vi "Distance elevation and azimuth calculation.vi"(0 "Julian Date":dbl, 2 "Antenna latitude (°)":dbl, 3 "Antenna east longitude (°)":dbl, 4 "Antenna altitude (km)":dbl, 5 "Position Satellite coordinate (ECI)":T1) -> (16 "Azimuth (deg)":dbl, 18 "Elevation (deg)":dbl)   [LabVIEW 2015]
uses:
  <vilib>/Analysis/Matrix/Datatypes/RealMatrix.ctl
  <vilib>/Analysis/Matrix/Numeric/Conversions/Matrix To Array - RM.vi
  Documents/LabVIEW Data/MathScriptVIs/MCStatic_35235434532_9082a658d9e3cba983ee0788969a3ccd.vi
  <instcachedir>/0/MCStatic_35235434532_9082a658d9e3cba983ee0788969a3ccd_E32396614517464C89ABB3D551BA75A9.lvgen/MCStatic_35235434532_9082a658d9e3cba983ee0788969a3ccd_E32396614517464C89ABB3D551BA75A9_000.vi
  Documents/LabVIEW Data/MathScriptVIs/MCStatic_35235434532_d6c4c3a44b84e4e53bab3d751e02fcec.vi
  <instcachedir>/0/MCStatic_35235434532_d6c4c3a44b84e4e53bab3d751e02fcec_188007D13E77446E935A379BA33C246C.lvgen/MCStatic_35235434532_d6c4c3a44b84e4e53bab3d751e02fcec_188007D13E77446E935A379BA33C246C_000.vi
  <vilib>/imath/engines/lvmath2/RunTimeEngine/IndexRead/NIMS V(S).vi
  <instcachedir>/0/NIMS V(S)_0488751826AF41519A22953C041130DC.lvgen/NIMS V(S)_0488751826AF41519A22953C041130DC_000.vi
  <vilib>/imathl/engines/lvmath/Functions/Error Handling/Create Error.vi
  <vilib>/imath/engines/lvmath2/RunTimeEngine/NodeEndStatement/NIMS_NodeEndStatement_Output.vi
  <instcachedir>/0/NIMS_NodeEndStatement_Output_53EC0D466D134D7ABD903AC30B43404B.lvgen/NIMS_NodeEndStatement_Output_53EC0D466D134D7ABD903AC30B43404B_001.vi
  <vilib>/imath/engines/lvmath2/RunTimeEngine/ErrorHandling/NIMS_Finalize Error.vi
  Matlab_codes/ECEFtoAzEl.m
  Matlab_codes/R2.m
  Matlab_codes/R3.m
  Matlab_codes/ECItoECEF.m
  Matlab_codes/JD2GAST.m
  Matlab_codes/JD2GMST.m
  Matlab_codes/MultiDimMatrixMultiply.m
  Matlab_codes/T3D.m
  <vilib>/Analysis/Matrix/NI_Matrix.lvlib
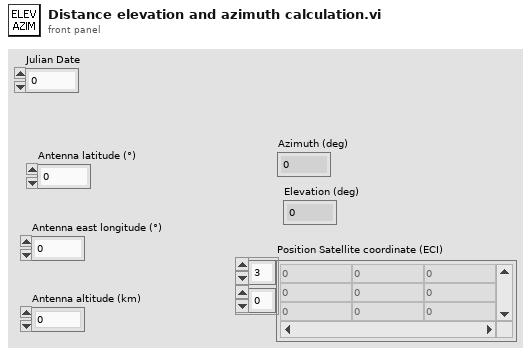
[diagram p1: front panel]
types:
  T1 = typedef "NI_Matrix.lvlib/RealMatrix.ctl" = dbl[][]
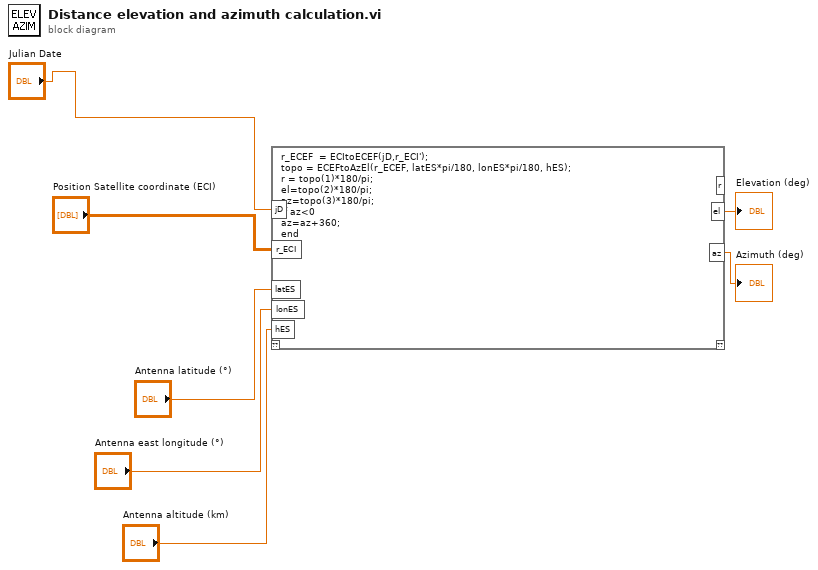
[diagram p0: block diagram]
diagram:
  n1 = mathscript code="r_ECEF  = ECItoECEF(jD,r_ECI');\ntopo = ECEFtoAzEl(r_ECEF, latES*pi/180, lonES*pi/180, hES);\nr = topo(1)*180/pi;\nel=topo(2)*180/pi;\naz=topo(3)*180/pi;\nif az<0\naz=az+360;\nend" ("Nœud MathScript")("jD"="Julian Date", "r_ECI"="Position Satellite coordinate (ECI)", "latES"="Antenna latitude (°)", "lonES"="Antenna east longitude (°)", "hES"="Antenna altitude (km)") -> ("el"=→"Elevation (deg)":dbl, "az"=→"Azimuth (deg)":dbl)  [unwired: 1 in, 2 out]
